vi "XML ( Get Node Value ).vi"   [LabVIEW 2018, in "XML.lvlib" / "XML.lvclass"]
uses:
  XML.lvclass
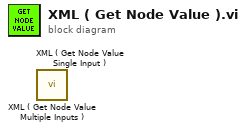
[diagram p0: block diagram]
diagram:
  n1 = call "XML ( Get Node Value Multiple Inputs ).vi"() -> ()  [unwired: 9 in, 3 out]
  n2 = call "XML ( Get Node Value Single Input ).vi"() -> ()  [unwired: 9 in, 3 out]
